vi "Template.vi"(8 "error in (no error)":errorcluster, 9 "Mode (Read / Write)":enum8{"Write", "Read"}(ring), 10 "Window (Hamming)":T1(ring)=enum."Hamming", 11 "telnet connection":T2) -> (0 "error out":errorcluster, 1 "Window?":T1(ring)=enum."Hamming", 2 "response data":string, 3 "telnet  connection out":T2)   [LabVIEW 2011]
doc: "Insight Photonic Solutions\n\nThis VI sets the Window used to calculate the FFT in Measurement Mode.\n\nver 1.0 - original release"
uses:
  Telnet Session.ctl
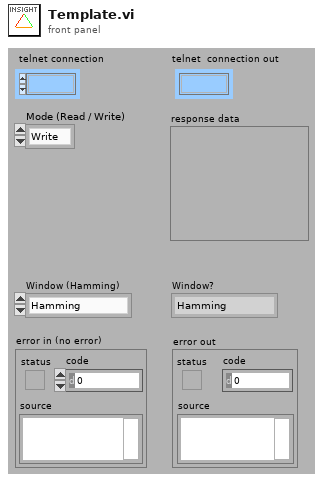
[diagram p1: front panel]
types:
  T1 = enum16{"No windowing", "Hann", "Hamming", "Blackman", "Blackman-Harris"}
  T2 = typedef "Telnet Session.ctl" = refnum<k1>
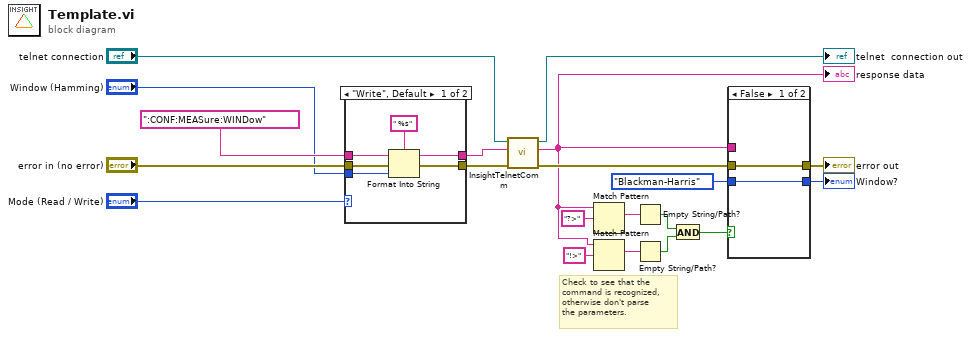
[diagram p0: block diagram]
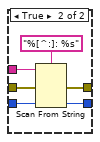
[diagram p2: hidden frame]
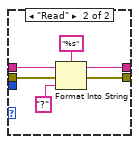
[diagram p3: hidden frame]
diagram:
  # "Check to see that the \ncommand is recognized,\notherwise don't parse \nthe parameters."
  n1 = case shown="\"Write\", Default" "Mode (Read / Write)" {
    tunnel: [w26 w28] -> w16
    tunnel: "error in (no error)" -> [w25 w27]
    tunnel: ":CONF:MEASure:WINDow" ("String") -> [w24 w30]
    tunnel: "Window (Hamming)" -> [w23 _]
    tunnel: [w21 w29] -> w14
    frame "Write", Default {
      n2 = Format Into String(format string=" %s", initial string=w24, error in=w25, w23) -> (resulting string=w21:string, error out=w26:errorcluster)
    }
    frame "Read" {
      n3 = Format Into String(format string="%s", initial string=w30, error in=w27, "?" ("input 1")) -> (resulting string=w29:string, error out=w28:errorcluster)
    }
  }
  n4 = call "InsightTelnetComm.vi"("error in"=w16, "write buffer (\"\")"=w14, "telnet connection"="telnet connection") -> ("error out"=w15:errorcluster, "response data"=w1:string, "telnet  connection out"=→"telnet  connection out":T2)  [unwired: 4 in]
  "response data" <- w1
  n5 = Match Pattern(string=w1, regular expression="?>") -> (match substring=w7:string)  [unwired: 1 in, 3 out]
  n6 = Match Pattern(string=w1, regular expression="!>") -> (match substring=w6:string)  [unwired: 1 in, 3 out]
  n7 = Empty String/Path?(string/path=w7) -> (empty?=w4:bool)
  n8 = Empty String/Path?(string/path=w6) -> (empty?=w3:bool)
  n9 = And(x=w4, y=w3) -> (x .and. y?=w2:bool)
  n10 = case shown="False" w2 {
    tunnel: [w33 w39] -> w17
    tunnel: w15 -> [w33 w38]
    tunnel: w1 -> [_ w37]
    tunnel: T1."Blackman-Harris" ("Window (Hamming)") -> [w34 w36]
    tunnel: [w34 w35] -> w9
    frame False {
    }
    frame True {
      n11 = Scan From String(format string="%[^:]: %s", input string=w37, error in=w38, default 2=w36) -> (error out=w39:errorcluster, output 2=w35:T1)  [unwired: 3 in, 2 out]
    }
  }
  "error out" <- w17
  "Window?" <- w9
